vi "CH_LM DisplayData2FormatScale.vi"(0 "Display Data":cluster{"Format ID":u8, "Scale ID":u8}) -> (1 "Format String":string, 2 "Scale Multiplier":dbl format="%#.1e")   [LabVIEW 2012, in "CH_LM.lvlib"]
doc: "This VI converts the Display Data IDs to Format String and Scale Multiplier."
uses:
  CH_LM.lvlib
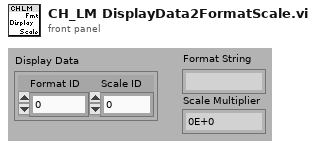
[diagram p1: front panel]
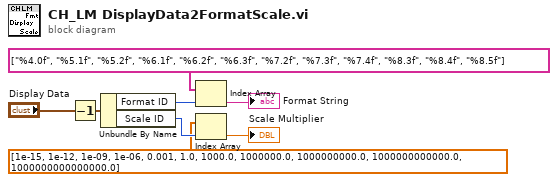
[diagram p0: block diagram]
diagram:
  n1 = Decrement(x="Display Data") -> (x-1=w7:cluster{"Format ID":u8, "Scale ID":u8})
  n2 = Unbundle By Name(w7) -> ("Format ID"=w6:u8, "Scale ID"=w5:u8)
  n3 = Index Array(array=string[] ["%4.0f", "%5.1f", "%5.2f", "%6.1f", "%6.2f", "%6.3f", "%7.2f", "%7.3f", "%7.4f", "%8.3f", "%8.4f", "%8.5f"], index=w6) -> (element=→"Format String":string)
  n4 = Index Array(array=dbl[] [1e-15, 1e-12, 1e-09, 1e-06, 0.001, 1.0, 1000.0, 1000000.0, 1000000000.0, 1000000000000.0, 1000000000000000.0], index=w5) -> (element=→"Scale Multiplier":dbl)
